vi "Actor Core.vi"(8 "error in":errorcluster, 11 "Fault Handler in":refnum<class "Fault Handler.lvclass">) -> (0 "error out":errorcluster, 3 "Actor out":refnum<class "Actor.lvclass">)   [LabVIEW 2023, in "Fault Handler.lvlib" / "Fault Handler.lvclass"]
doc: "<b>Bottom Panel</b> actor is an abstraction that provides the actor framework panel size definitions.\n\n<b>Fault Handler</b> This override implements the fault monitor software. \n\n<b> Events </b>\n\n1. Waits for a fault event to be triggered (Events generated by <b>Engine:Check For Errors</b> called consistently through the software. When an event is triggered, the software calls <b> Process Warning</b> or <b>Process Error</b> based on the Status bit of the error cluster.\n\n2. Monitors the Automation Reference Event (generated by <b>Engine:Send Automation Reference</b>) if a reference is provided, the software stores the reference in to private data so the fault handler has the capability of generating faults on the automated software.\n\n<b>User Events</b>\n\n1. After warnings and faults are dealt with, the fault records are cleared by operator intervention clicking clear alarms or clear warnings. \n\n2. The operator can also trigger a hide faults panel action which calls <b>Send Toggle Display</b> routine"
uses:
  Library/Fault Handler.lvclass
  C:/Users/Public/Documents/Development/builds/Engine/Engine.lvlibp/Project/Engine.lvclass
  builds/Engine/Actor Framework.lvlibp/1abvi3w/vi.lib/ActorFramework/Actor/Actor.lvclass
  Library/Fault Handler.lvclass/Fault Handler.ctl
  Accessors/Write Active Alarms.vi
  Accessors/Write Active Warnings.vi
  Accessors/Write Alarm Log.vi
  Accessors/Write Warning Log.vi
  builds/Engine/Engine.lvlibp/Accessors/Write VI_Ref.vi
  builds/Base Software/Panels/Bottom Panel.lvlibp/Project/Bottom.lvclass
panel:
  out "Warnings Log":string
  out "Active Warnings":i32(listbox)
  out "Alarm Log":string
  out "Active Alarms":i32(listbox)
  in  "Hide Faults":bool
  in  "Clear Alarms":bool
  in  "Clear Warnings":bool
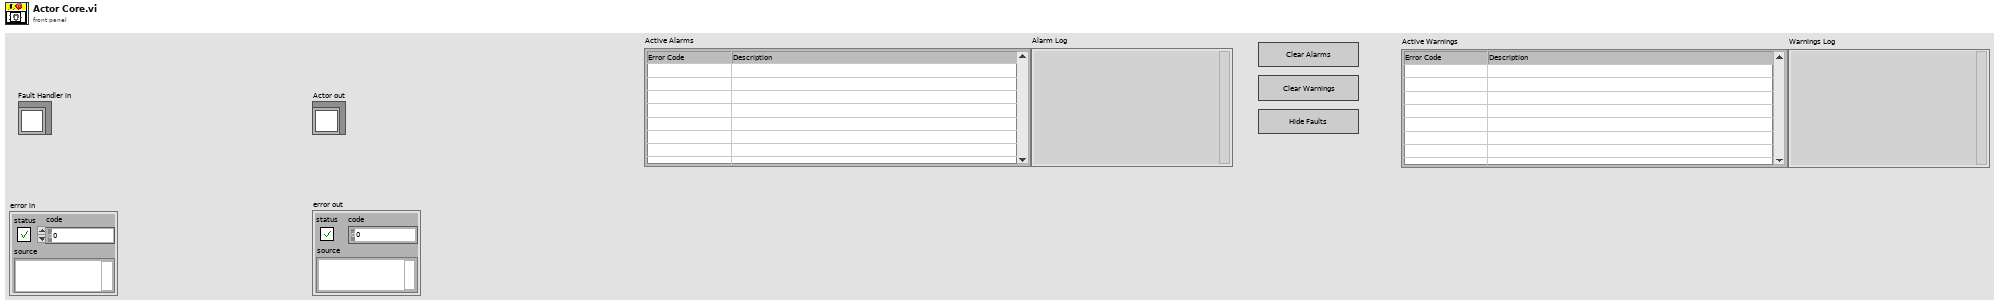
[diagram p1: front panel]
types:
  T1 = cluster{"Pnl Actor":refnum<event-registration>, "Event Registration Refnum":refnum<event-registration>}
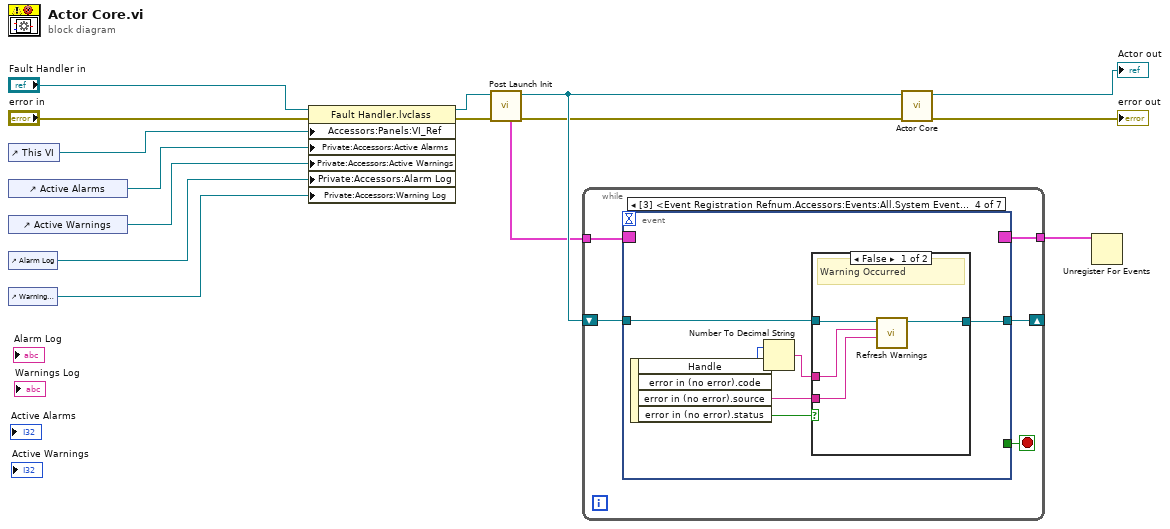
[diagram p0: block diagram]
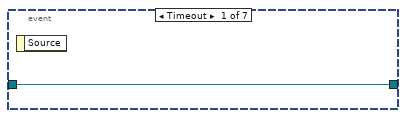
[diagram p2: hidden frame]
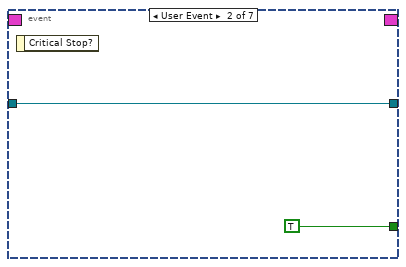
[diagram p3: hidden frame]
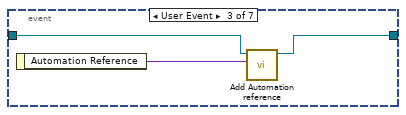
[diagram p4: hidden frame]
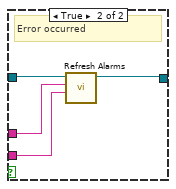
[diagram p5: hidden frame]
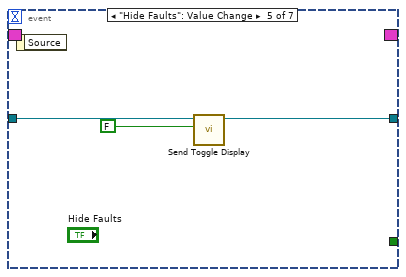
[diagram p6: hidden frame]
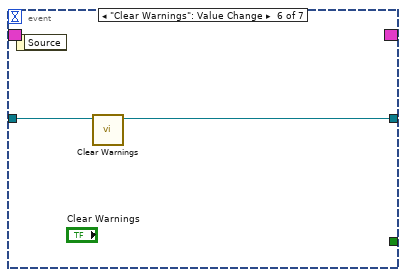
[diagram p7: hidden frame]
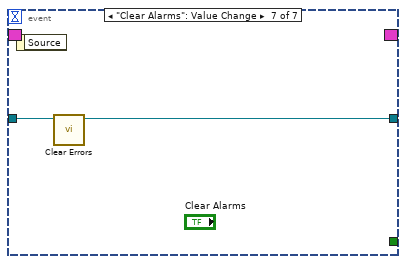
[diagram p8: hidden frame]
diagram:
  n1 = control-ref of="This VI"() -> (w11:refnum<vi>)
  n2 = control-ref of="Active Alarms"() -> (w4:refnum<vi>)
  n3 = control-ref of="Active Warnings"() -> (w3:refnum<vi>)
  n4 = control-ref of="Alarm Log"() -> (w2:refnum<vi>)
  n5 = control-ref of="Warnings Log"() -> (w1:refnum<vi>)
  n6 = property class="Fault Handler.lvclass"(reference="Fault Handler in", error in="error in", "Accessors:Panels:VI_Ref"=w11, "Private:Accessors:Active Alarms"=w4, "Private:Accessors:Active Warnings"=w3, "Private:Accessors:Alarm Log"=w2, "Private:Accessors:Warning Log"=w1) -> (reference out=w8:refnum<class "Fault Handler.lvclass">, error out=w9:errorcluster)
  n7 = call "Post Launch Init.vi"("error in"=w9, "Fault Handler in"=w8) -> ("error out"=w6:errorcluster, "Fault Handler out"=w7:refnum<class "Fault Handler.lvclass">, "Events"=w5:T1)  [unwired: 7 in]
  n8 = while {
    tunnel: w5 -> [w20]
    tunnel: [w19] -> w10
    shift-right: [w16] -> _
    shift-left: w7 -> [w17]
    stop <- w18 stop-if-true
    n9 = event shown="[3] <Event Registration Refnum.Accessors:Events:All.System Event.Fault Event>: User Event" {
      selector: w20 -> [_ _ _ _ _ _ _]
      dyn-events: [_ _ _ _ _ _ _] -> w19
      timeout: _ -> [_ _ _ _ _ _ _]
      tunnel: [_ TRUE _ _ _ _ _] -> w18
      tunnel: w17 -> [w21 w22 w26 w31 w43 w45 w47]
      tunnel: [w21 w22 w24 w27 w41 w44 w46] -> w16
      event Timeout {
        n10 = event-data() -> ()  [unwired: 1 in, 1 out]
      }
      event User Event {
        n11 = event-data() -> ()  [unwired: 1 in, 1 out]
      }
      event User Event {
        n12 = event-data() -> ("Automation Reference"=w25:variant)  [unwired: 1 in]
        n13 = call "Add Automation reference.vi"("Automation"=w25, "Fault Handler in"=w26) -> ("Fault Handler out"=w24:refnum<class "Fault Handler.lvclass">)  [unwired: 8 in, 1 out]
      }
      event User Event {
        n14 = event-data() -> ("error in (no error).code"=w28:i32, "error in (no error).source"=w32:string, "error in (no error).status"=w30:bool)  [unwired: 1 in, 1 out]
        n15 = Number To Decimal String(number=w28) -> (decimal integer string=w29:string)  [unwired: 1 in]
        n16 = case shown="False" w30 {
          tunnel: w32 -> [w34 w39]
          tunnel: w31 -> [w36 w40]
          tunnel: w29 -> [w35 w38]
          tunnel: [w33 w37] -> w27
          frame False {
            # "Warning Occurred"
            n17 = call "Refresh Warnings.vi"("Source"=w34, "Code"=w35, "Fault Handler in"=w36) -> ("Fault Handler out"=w33:refnum<class "Fault Handler.lvclass">)  [unwired: 7 in, 1 out]
          }
          frame True {
            # "Error occurred"
            n18 = call "Refresh Alarms.vi"("Source"=w39, "Code"=w38, "Fault Handler in"=w40) -> ("Fault Handler out"=w37:refnum<class "Fault Handler.lvclass">)  [unwired: 7 in, 1 out]
          }
        }
      }
      event "Hide Faults": Value Change {
        n19 = event-data() -> ()  [unwired: 1 in, 1 out]
        n20 = call "Send Toggle Display.vi"("Show"=FALSE, "Fault Handler in"=w43) -> ("Fault Handler out"=w41:refnum<class "Fault Handler.lvclass">)  [unwired: 8 in, 1 out]
      }
      event "Clear Warnings": Value Change {
        n21 = event-data() -> ()  [unwired: 1 in, 1 out]
        n22 = call "Clear Warnings.vi"("Fault Handler in"=w45) -> ("Fault Handler out"=w44:refnum<class "Fault Handler.lvclass">)  [unwired: 9 in, 1 out]
      }
      event "Clear Alarms": Value Change {
        n23 = event-data() -> ()  [unwired: 1 in, 1 out]
        n24 = call "Clear Errors.vi"("Fault Handler in"=w47) -> ("Fault Handler out"=w46:refnum<class "Fault Handler.lvclass">)  [unwired: 9 in, 1 out]
      }
    }
  }
  n25 = call-parent "Actor Core.vi"("error in"=w6, "Bottom in"=w7) -> ("error out"=→"error out":errorcluster, "Actor out"=→"Actor out":refnum<class "Actor.lvclass">)  [unwired: 8 in]
  n26 = Unregister For Events(event registration refnum=w10) -> ()  [unwired: 1 in, 1 out]
